vi "Refactor Dependencies for Project.vi"(8 "error in (no error)":errorcluster, 10 "refactor data":T6, 11 "project path":path) -> (0 "error out":errorcluster, 2 "refactor result":T1)   [LabVIEW 2020, in "MeasurementService Editor.lvlib"]
uses:
  MeasurementService Editor.lvlib
  Rename Refactor Data.ctl
  Rename Refactor Mapping Info.ctl
  Rename String Mapping.ctl
  Refactor Project Result.ctl
  Refactor Object Result.ctl
  Refactor Dynamic Dispatch Member Result.ctl
  Rename String Result.ctl
  Rename String.ctl
panel:
  out "items processed":i32
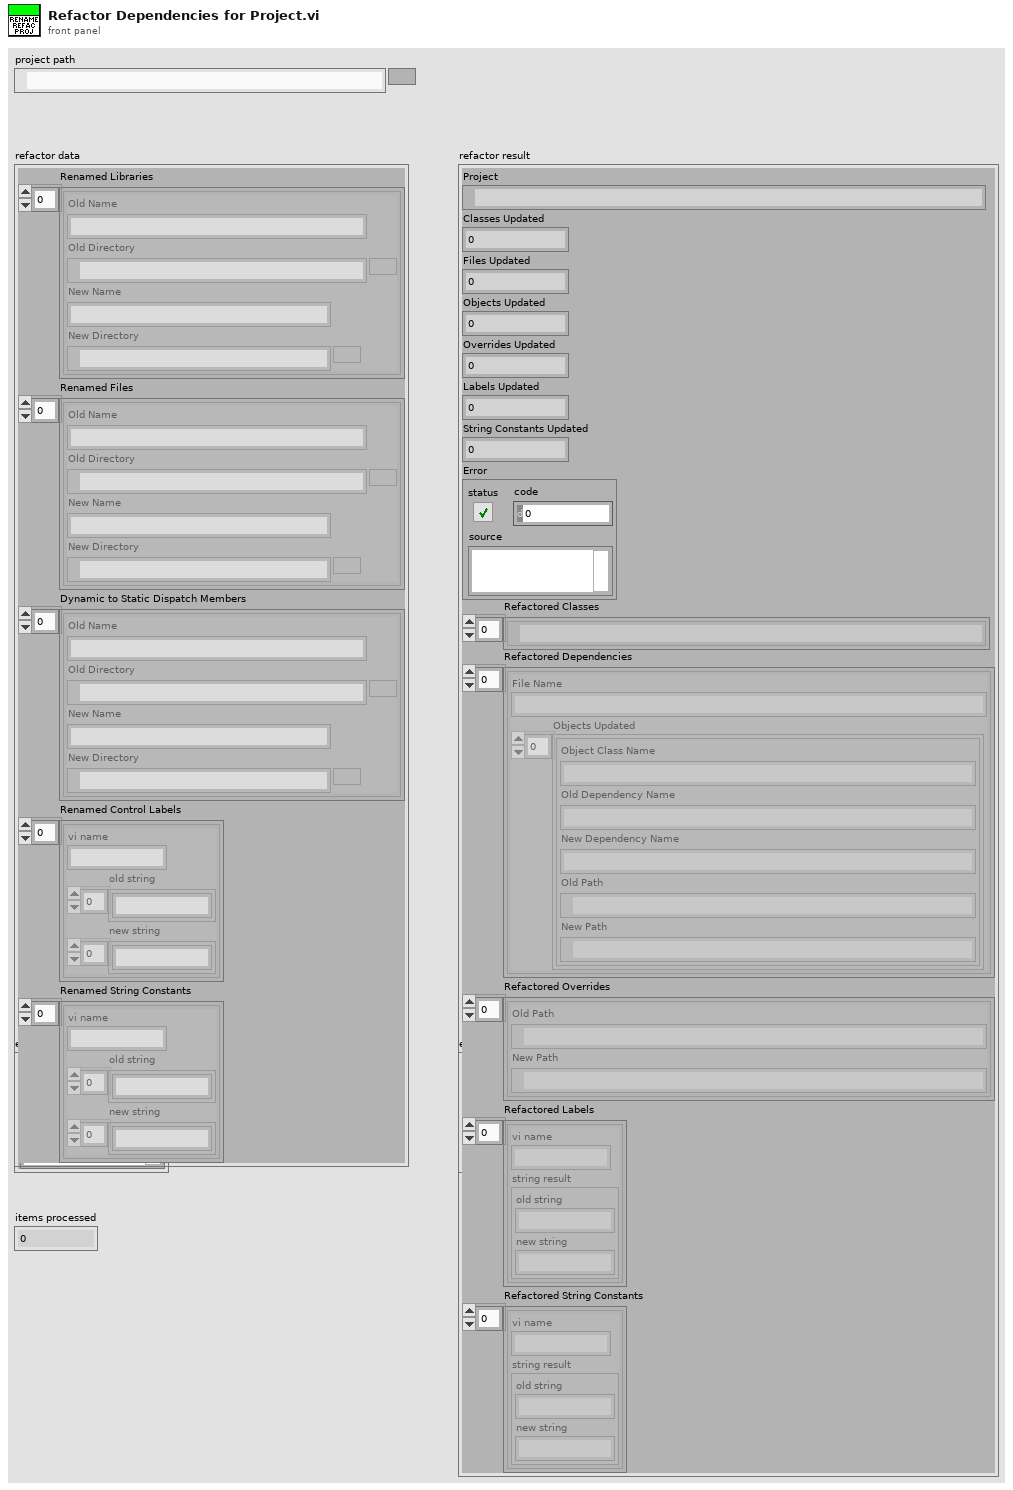
[diagram p1: front panel]
types:
  T1 = typedef "MeasurementService Editor.lvlib/Refactor Project Result.ctl" = cluster{"Project":path, "Classes Updated":u32, "Files Updated":u32, "Objects Updated":u32, "Overrides Updated":u32, "Labels Updated":u32, "String Constants Updated":u32, "Error":errorcluster, "Refactored Classes":path[], "Refactored Dependencies":cluster{"File Name":string, "Objects Updated":T2[]}[], "Refactored Overrides":T3[], "Refactored Labels":T4[], "Refactored String Constants":T4[]}
  T2 = typedef "MeasurementService Editor.lvlib/Refactor Object Result.ctl" = cluster{"Object Class Name":string, "Old Dependency Name":string, "New Dependency Name":string, "Old Path":path, "New Path":path}
  T3 = typedef "MeasurementService Editor.lvlib/Refactor Dynamic Dispatch Member Result.ctl" = cluster{"Old Path":path, "New Path":path}
  T4 = typedef "MeasurementService Editor.lvlib/Rename String Result.ctl" = cluster{"vi name":string, "string result":T5}
  T5 = typedef "MeasurementService Editor.lvlib/Rename String.ctl" = cluster{"old string":string, "new string":string}
  T6 = typedef "MeasurementService Editor.lvlib/Rename Refactor Data.ctl" = cluster{"Renamed Libraries":T7[], "Renamed Files":T7[], "Dynamic to Static Dispatch Members":T7[], "Renamed Control Labels":T8[], "Renamed String Constants":T8[]}
  T7 = typedef "MeasurementService Editor.lvlib/Rename Refactor Mapping Info.ctl" = cluster{"Old Name":string, "Old Directory":path, "New Name":string, "New Directory":path}
  T8 = typedef "MeasurementService Editor.lvlib/Rename String Mapping.ctl" = cluster{"vi name":string, "old string":string[], "new string":string[]}
  T9 = cluster{"File Name":string, "Objects Updated":T2[]}
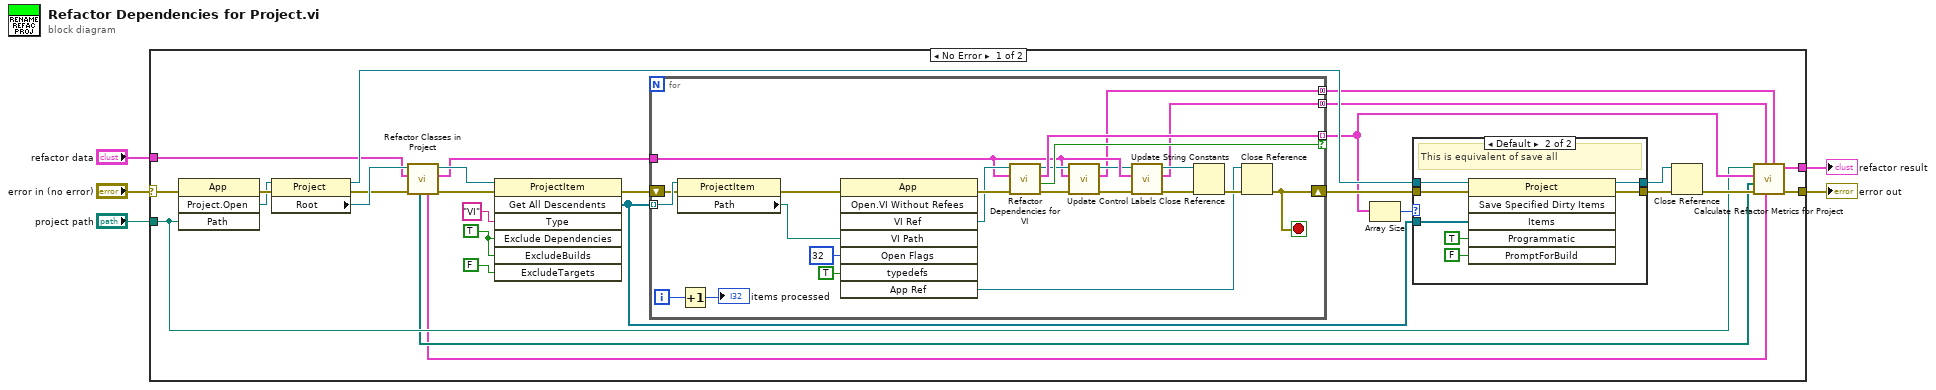
[diagram p0: block diagram]
diagram:
  n1 = case shown="No Error" "error in (no error)" {
    selector: "error in (no error)" -> [w17 w67]
    tunnel: "project path" -> [w11 _]
    tunnel: [w14 w67] -> w4
    tunnel: "refactor data" -> [w18 _]
    tunnel: [w13 _] -> w1
    frame No Error {
      w33 = TRUE ("ExcludeDependencies")
      n2 = invoke class="App" method="Project.Open"(error in=w17, "Path"=w11) -> (error out=w31:errorcluster, "Project:Open"=w30:refnum<vi>)  [unwired: 2 in, 2 out]
      n3 = property class="Project"(reference=w30, error in=w31) -> (reference out=w22:refnum<vi>, error out=w20:errorcluster, "Root"=w21:refnum<vi>)
      n4 = call "Refactor Classes in Project.vi"("error in (no error)"=w20, "rename data in"=w18, "project item in"=w21) -> ("error out"=w19:errorcluster, "rename metadata out"=w8:T6, "project item out"=w16:refnum<vi>, "refactored overrides"=w9:T3[], "refactored classes"=w10:path[])  [unwired: 4 in]
      n5 = invoke class="ProjectItem" method="Get All Descendents"(reference=w16, error in=w19, "Type"="VI", "Exclude Dependencies"=w33, "ExcludeBuilds"=w33, "ExcludeTargets"=FALSE) -> (error out=w29:errorcluster, "All Descendents"=w23:refnum<vi>[])  [unwired: 1 in, 5 out]
      n6 = for {
        tunnel: w23 -> [w57] mode=indexing
        shift-right: [w38] -> w26
        shift-left: w29 -> [w56]
        tunnel: [w51] -> w12 mode=indexing if=w55
        tunnel: w8 -> [w42]
        tunnel: [w35] -> w7 mode=concatenating
        tunnel: [w34] -> w6 mode=concatenating
        i -> [w54]
        stop <- w38 stop-if-true
        n7 = property class="ProjectItem"(reference=w57, error in=w56) -> (error out=w47:errorcluster, "Path"=w46:path)  [unwired: 1 out]
        n8 = Increment(x=w54) -> (x+1=→"items processed":i32)
        n9 = invoke class="App" method="Open.VI Without Refees"(error in=w47, "VI Path"=w46, "Open Flags"=32 ("options"), "typedefs"=TRUE ("Load Typedefs?")) -> (error out=w45:errorcluster, "VI Ref"=w44:refnum<vi>, "App Ref"=w36:refnum<vi>)  [unwired: 4 in, 5 out]
        n10 = call "Refactor Dependencies for VI.vi"("error in"=w45, "rename data"=w42, "vi reference in"=w44) -> ("error out"=w52:errorcluster, "missing dependencies"=w55:bool, "missing items"=w51:T9, "vi reference out"=w43:refnum<vi>)  [unwired: 5 in]
        n11 = call "Update Control Labels.vi"("error in"=w52, "rename data"=w42, "vi reference in"=w43) -> ("error out"=w50:errorcluster, "rename labels result"=w35:T4[], "vi reference out"=w41:refnum<vi>)  [unwired: 6 in]
        n12 = call "Update String Constants.vi"("error in"=w50, "rename data"=w42, "vi reference in"=w41) -> ("error out"=w40:errorcluster, "rename string constants results"=w34:T4[], "vi reference out"=w37:refnum<vi>)  [unwired: 6 in]
        n13 = Close Reference(reference=w37, error in (no error)=w40) -> (error out=w39:errorcluster)
        n14 = Close Reference(reference=w36, error in (no error)=w39) -> (error out=w38:errorcluster)
      }
      n15 = Array Size(array=w12) -> (size(s)=w24:i32)
      n16 = case shown="Default" w24 {
        tunnel: w22 -> [w58 w66]
        tunnel: [w58 w60] -> w27
        tunnel: w26 -> [w59 w65]
        tunnel: [w59 w64] -> w25
        tunnel: w23 -> [_ w63]
        frame 0 {
        }
        frame Default {
          # "This is equivalent of save all"
          n17 = invoke class="Project" method="Save Specified Dirty Items"(reference=w66, error in=w65, "Items"=w63, "Programmatic"=TRUE, "PromptForBuild"=FALSE) -> (reference out=w60:refnum<vi>, error out=w64:errorcluster)  [unwired: 1 in, 4 out]
        }
      }
      n18 = Close Reference(reference=w27, error in (no error)=w25) -> (error out=w15:errorcluster)
      n19 = call "Calculate Refactor Metrics for Project.vi"("refactored labels"=w7, "refactored overrides"=w9, "refactored string constants"=w6, "error in"=w15, "refactored classes"=w10, "refactored dependencies"=w12, "project path"=w11) -> ("error out"=w14:errorcluster, "refactor result"=w13:T1)  [unwired: 3 in]
    }
    frame Error {
    }
  }
  "error out" <- w4
  "refactor result" <- w1
